vi "SetCMYK.vi"(0 "ColorRGB in":refnum<class "ColorCMYK.lvclass">, 5 "C (%)":dbl, 7 "M (%)":dbl, 9 "Y (%)":dbl, 11 "error in (no error)":errorcluster, 12 "K (%)":dbl) -> (4 "ColorRGB out":refnum<class "ColorCMYK.lvclass">, 15 "error out":errorcluster)   [LabVIEW 2021, in "Picture2D.lvlib" / "ColorCMYK.lvclass"]
uses:
  ColorCMYK.lvclass
  ColorCMYK.lvclass/ColorCMYK.ctl
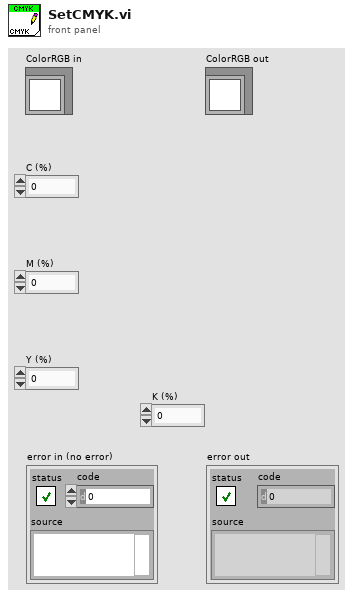
[diagram p1: front panel]
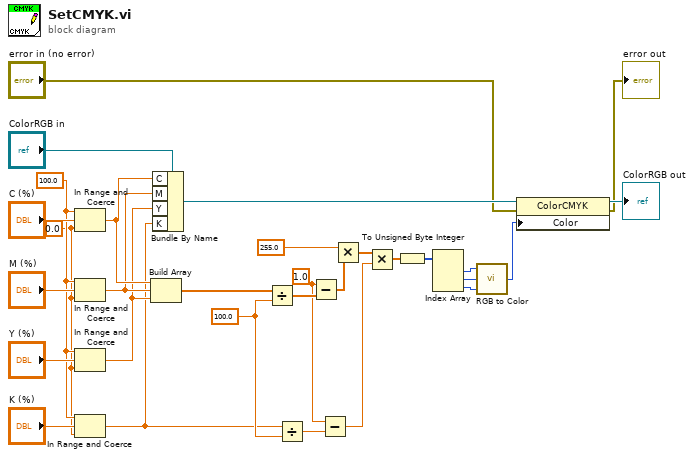
[diagram p0: block diagram]
diagram:
  w1 = 0.0 ("lower limit")
  w2 = 100.0 ("upper limit")
  w15 = 1.0
  w19 = 100.0
  n1 = In Range and Coerce(upper limit=w2, x="C (%)", lower limit=w1) -> (coerced(x)=w6:dbl)  [unwired: 1 out]
  n2 = In Range and Coerce(upper limit=w2, x="M (%)", lower limit=w1) -> (coerced(x)=w5:dbl)  [unwired: 1 out]
  n3 = In Range and Coerce(upper limit=w2, x="Y (%)", lower limit=w1) -> (coerced(x)=w4:dbl)  [unwired: 1 out]
  n4 = In Range and Coerce(upper limit=w2, x="K (%)", lower limit=w1) -> (coerced(x)=w3:dbl)  [unwired: 1 out]
  n5 = Build Array(w6, w5, w4) -> (w24:dbl[])
  n6 = Bundle By Name(cluster="ColorRGB in", "C"=w6, "M"=w5, "Y"=w4, "K"=w3) -> (w29:refnum<class "ColorCMYK.lvclass">)
  n7 = Divide(x=w24, y=w19) -> (x/y=w22:dbl[])
  n8 = Divide(x=w3, y=w19) -> (x/y=w17:dbl)
  n9 = Subtract(x=w15, y=w22) -> (x-y=w21:dbl[])
  n10 = Subtract(x=w15, y=w17) -> (x-y=w16:dbl)
  n11 = Multiply(x=255.0, y=w21) -> (x*y=w18:dbl[])
  n12 = Multiply(x=w18, y=w16) -> (x*y=w14:dbl[])
  n13 = To Unsigned Byte Integer(number=w14) -> (unsigned 8bit integer=w12:u8[])
  n14 = Index Array(array=w12) -> (element #1=w13:u8, element #2=w11:u8, element #3=w10:u8)  [unwired: 3 in]
  n15 = call <vilib>:"RGB to Color.vi"("B"=w10, "G"=w11, "R"=w13) -> ("Color"=w28:u32)
  n16 = property class="ColorCMYK"(reference=w29, error in="error in (no error)", "Color"=w28) -> (reference out=→"ColorRGB out":refnum<class "ColorCMYK.lvclass">, error out=→"error out":errorcluster)
